vi "Shutter Swing V3.vi"(6 "Retry #":i32=3, 9 "Shutter Drive":tag="Log/ao0", 10 "Damping":bool, 11 "Shutter close":bool) -> (0 "error out":errorcluster, 1 "Shutter close fdbk":bool, 2 "Fail #":u8, 3 "SEM shutter status":string, 4 "SDev":sgl format="%.4f", 5 "Color Box":u32(colorbox), 7 "Specimen I Graph":dbl[](graph))   [LabVIEW 2018]
uses:
  <vilib>/gmath/NI_Gmath.lvlib
panel:
  out "thresh":dbl
  out "SDev > Thresh?":bool
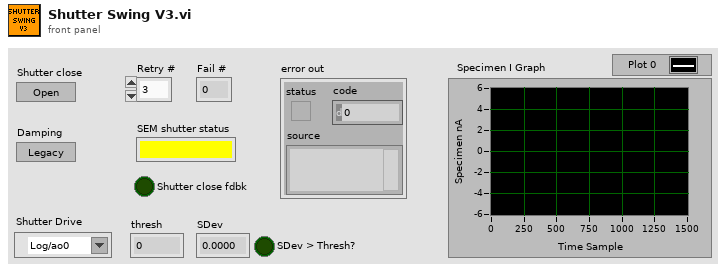
[diagram p1: front panel]
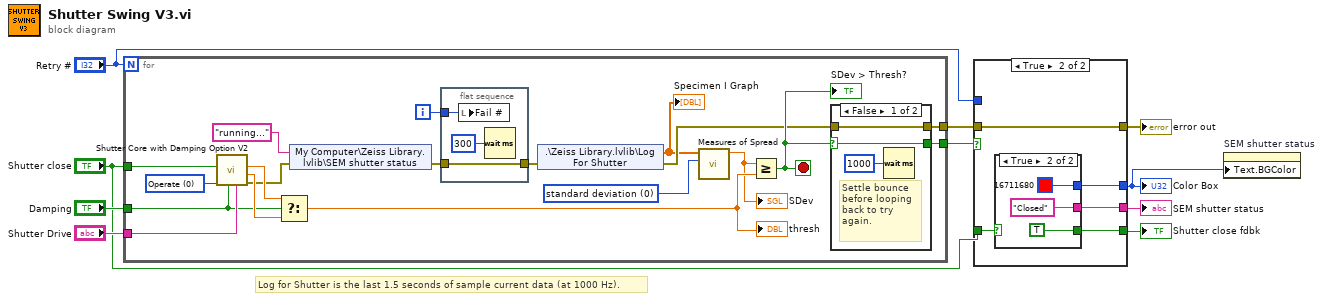
[diagram p0: block diagram]
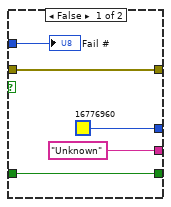
[diagram p2: hidden frame]
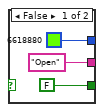
[diagram p3: hidden frame]
diagram:
  # "Log for Shutter is the last 1.5 seconds of sample current data (at 1000 Hz)."
  n1 = for {
    N: "Retry #" -> [_]
    tunnel: "Shutter Drive" -> [w29]
    tunnel: "Shutter close" -> [w28]
    tunnel: "Damping" -> [w17]
    tunnel: [w24] -> w6
    tunnel: [w22] -> w4
    i -> [w21]
    stop <- w25 stop-if-true
    w16 = u16 0 items=["Operate", "Initialize", "Read from .INI", "Write to .INI"] ("Action")
    w26 = 0 items=["standard deviation", "range", "mean absolute deviation", "interquartile range"] ("type")
    n2 = call "Shutter Core with Damping Option V2.vi"("Shutter Drive"=w29, "Damping"=w17, "Action"=w16, "OPEN-CLOSE"=w28) -> ("error out"=w12:errorcluster, "Legacy thrsh (nA)"=w19:dbl, "Damped thrsh (nA)"=w20:dbl)  [unwired: 4 in, 1 out]
    n3 = Select(t=w20, s=w17, f=w19) -> (s? t:f=w23:dbl)
    "thresh" <- w23
    n4 = shared-variable "My Computer\\Zeiss Library.lvlib\\SEM shutter status"("running..." ("SEM shutter status"), error in=w12) -> (error out=w13:errorcluster)
    n5 = flat-sequence {
      tunnel: w13 -> [w37]
      tunnel: [w37] -> w27
      tunnel: w21 -> [w36]
      frame #0 {
        n6 = local write "Fail #"(w36) -> ()
        n7 = Wait (ms)(milliseconds to wait=u32 300) -> ()  [unwired: 1 out]
      }
    }
    n8 = shared-variable ".\\Zeiss Library.lvlib\\Log For Shutter"(error in=w27) -> (w11:dbl[], error out=w14:errorcluster)
    "Specimen I Graph" <- w11
    n9 = call <vilib>:"Measures of Spread.vi"("type"=w26, "x array"=w11) -> ("spread value"=w15:dbl)  [unwired: 8 in, 1 out]
    "SDev" <- w15
    n10 = Greater Or Equal?(x=w15, y=w23) -> (x >= y?=w25:bool)
    "SDev > Thresh?" <- w25
    n11 = case shown="False" w25 {
      selector: w25 -> [w30 w33]
      tunnel: w14 -> [w31 w34]
      tunnel: [w31 w34] -> w24
      tunnel: [w30 w33] -> w22
      frame False {
        # "Settle bounce\nbefore looping\nback to try \nagain."
        n12 = Wait (ms)(milliseconds to wait=u32 1000) -> ()  [unwired: 1 out]
      }
      frame True {
      }
    }
  }
  n13 = case shown="True" w4 {
    tunnel: ["Unknown" w47] -> w8
    tunnel: "Retry #" -> [w39 _]
    tunnel: [w41 w46] -> w7
    tunnel: "Shutter close" -> [w41 w45]
    tunnel: w6 -> [w40 w44]
    tunnel: [w40 w44] -> w5
    tunnel: [u32 16776960 w43] -> w1
    frame False {
      "Fail #" <- w39
    }
    frame True {
      n14 = case shown="True" w45 {
        tunnel: ["Open" "Closed"] -> w47
        tunnel: [FALSE ("Shutter close") TRUE ("Shutter close")] -> w46
        tunnel: [u32 6618880 u32 16711680] -> w43
        frame False {
        }
        frame True {
        }
      }
    }
  }
  "SEM shutter status" <- w8
  "error out" <- w5
  "Shutter close fdbk" <- w7
  "Color Box" <- w1
  n15 = property on="SEM shutter status" class="Str"("Text.BGColor"=w1) -> ()  [unwired: 2 in, 2 out]
